vi "Set Pin Simulated.vi"(11 "Command to Send":string="SRC012;") -> (1 "Pin":bool, 2 "Valor Pin":string, 3 "Puerto":string)   [LabVIEW 2020, in "UI Actor.lvlib" / "UI Actor.lvclass"]
uses:
  UI Actor.lvclass
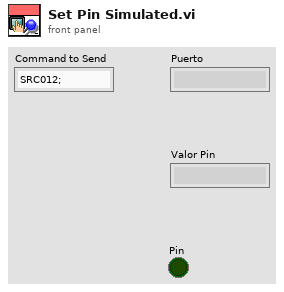
[diagram p1: front panel]
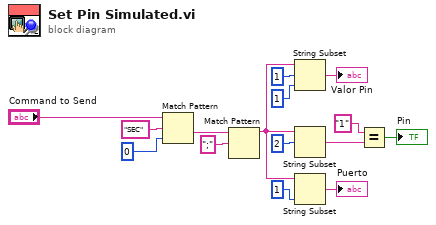
[diagram p0: block diagram]
diagram:
  n1 = Match Pattern(string="Command to Send", regular expression="SEC" ("string"), offset (0)=0) -> (after substring=w12:string)  [unwired: 3 out]
  n2 = Match Pattern(string=w12, regular expression=";") -> (before substring=w4:string)  [unwired: 1 in, 3 out]
  n3 = String Subset(string=w4, offset (0)=1, length (rest)=1 ("length (rest)")) -> (substring=→"Valor Pin":string)
  n4 = String Subset(string=w4, offset (0)=2) -> (substring=w7:string)  [unwired: 1 in]
  n5 = String Subset(string=w4, length (rest)=1 ("length (rest)")) -> (substring=→"Puerto":string)  [unwired: 1 in]
  n6 = Equal?(x="1", y=w7) -> (x = y?=→"Pin":bool)
